vi "Test.vi"   [LabVIEW 2017]
doc: "This VI is called when test mode begins, and will automatically be terminated when it ends. You can add manual or automatic tests and invoke them from the dashboard."
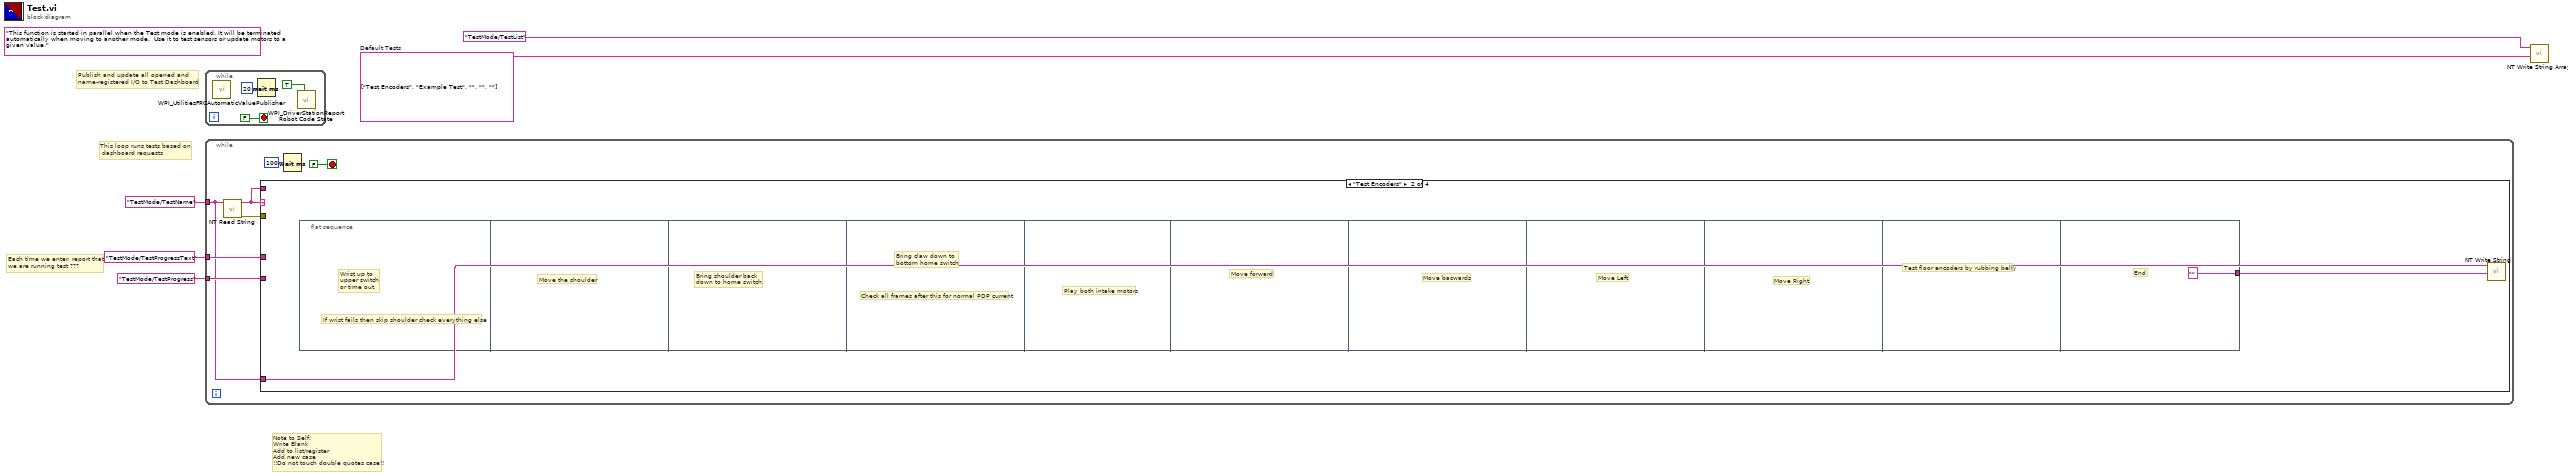
[diagram p0: block diagram]
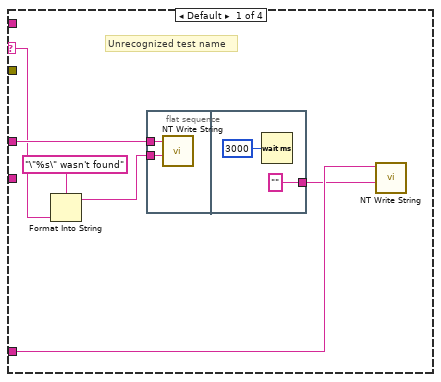
[diagram p2: hidden frame]
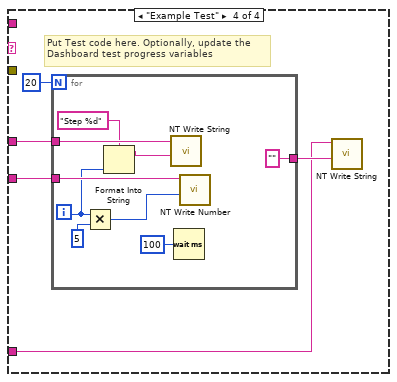
[diagram p4: hidden frame]
diagram:
  w2 = string[] ["Test Encoders", "Example Test", "", "", ""]  # Default Tests
  (unwired) "This function is started in parallel when the Test mode is enabled. It will be terminated automatically when moving to another mode.  Use it to test sensors or update motors to a given value."
  # "Note to Self:\nWrite Blank\nAdd to list/register\nAdd new case\n!!Do not touch double quotes case!!"
  # "This loop runs tests based on \n dashboard requests"
  # "Publish and update all opened and\nname-registered I/O to Test Dashboard"
  # "Each time we enter, report that\nwe are running test ???"
  n1 = while {
    stop <- FALSE stop-if-true
    n2 = call <vilib>:"WPI_UtilitiesFRCAutomaticValuePublisher.vi"() -> ()  [unwired: 12 in]
    n3 = Wait (ms)(milliseconds to wait=u32 20) -> ()  [unwired: 1 out]
    n4 = call <vilib>:"WPI_DriverStationReport Robot Code State.vi"("Test"=TRUE ("Autonomous")) -> ()  [unwired: 10 in, 1 out]
  }
  n5 = while {
    tunnel: "TestMode/TestName" ("Name") -> [w10]
    tunnel: "TestMode/TestProgressText" ("Name") -> [w13]
    tunnel: "TestMode/TestProgress" ("Name") -> [w12]
    stop <- FALSE stop-if-true
    n6 = call <vilib>:"NT Read String.vi"("Name"=w10) -> ("error out"=w9:errorcluster, "String"=w11:string)  [unwired: 9 in]
    n7 = case shown="\"Test Encoders\"" w11 {
      selector: w11 -> [w20 _ _ _]
      tunnel: w10 -> [w17 w27 _ w29]
      tunnel: w13 -> [w21 _ _ w32]
      tunnel: w12 -> [_ _ _ w33]
      tunnel: w11 -> [_ _ _ _]
      tunnel: w9 -> [_ _ _ _]
      frame Default {
        # "Unrecognized test name"
        n8 = Format Into String(format string="\"%s\" wasn't found" ("Name"), w20) -> (resulting string=w19:string)  [unwired: 2 in, 1 out]
        n9 = flat-sequence {
          tunnel: w21 -> [w22]
          tunnel: w19 -> [w23]
          tunnel: ["" ("Name")] -> w16
          frame #0 {
            n10 = call <vilib>:"NT Write String.vi"("String"=w23, "Name"=w22) -> ()  [unwired: 9 in, 1 out]
          }
          frame #1 {
            n11 = Wait (ms)(milliseconds to wait=u32 3000) -> ()  [unwired: 1 out]
          }
        }
        n12 = call <vilib>:"NT Write String.vi"("String"=w16, "Name"=w17) -> ()  [unwired: 9 in, 1 out]
      }
      frame "Test Encoders" {
        n13 = flat-sequence {
          tunnel: ["" ("String")] -> w26
          frame #0 {
            # "If wrist fails then skip shoulder check everything else"
            # "Wrist up to \nupper switch\nor time out"
          }
          frame #1 {
            # "Move the shoulder"
          }
          frame #2 {
            # "Bring shoulder back \ndown to home switch"
          }
          frame #3 {
            # "Check all frames after this for normal PDP current"
            # "Bring claw down to\nbottom home switch"
          }
          frame #4 {
            # "Play both intake motors"
          }
          frame #5 {
            # "Move forward"
          }
          frame #6 {
            # "Move bacwards"
          }
          frame #7 {
            # "Move Left"
          }
          frame #8 {
            # "Move Right"
          }
          frame #9 {
            # "Test floor encoders by rubbing belly"
          }
          frame #10 {
            # "End"
          }
        }
        n14 = call <vilib>:"NT Write String.vi"("String"=w26, "Name"=w27) -> ()  [unwired: 9 in, 1 out]
      }
      frame "" {
      }
      frame "Example Test" {
        # "Put Test code here. Optionally, update the\nDashboard test progress variables"
        n15 = for {
          N: 20 -> [_]
          tunnel: w33 -> [w42]
          tunnel: w32 -> [w40]
          tunnel: ["" ("String")] -> w30
          i -> [w37]
          n16 = Multiply(x=w37, y=u32 5 ("milliseconds to wait")) -> (x*y=w38:u32)
          n17 = Format Into String(format string="Step %d", w37) -> (resulting string=w35:string)  [unwired: 2 in, 1 out]
          n18 = call <vilib>:"NT Write String.vi"("String"=w35, "Name"=w40) -> ()  [unwired: 9 in, 1 out]
          n19 = Wait (ms)(milliseconds to wait=u32 100) -> ()  [unwired: 1 out]
          n20 = call <vilib>:"NT Write Number.vi"("Numeric"=w38, "Name"=w42) -> ()  [unwired: 9 in, 1 out]
        }
        n21 = call <vilib>:"NT Write String.vi"("String"=w30, "Name"=w29) -> ()  [unwired: 9 in, 1 out]
      }
    }
    n22 = Wait (ms)(milliseconds to wait=u32 100) -> ()  [unwired: 1 out]
  }
  n23 = call <vilib>:"NT Write String Array.vi"("String Array"=w2, "Name"="TestMode/TestList") -> ()  [unwired: 9 in, 1 out]
